vi "Initialise.vi"(8 "error in (no error)":errorcluster, 10 "Var Access":refnum<class "Var_Access.lvclass">[](array[class]), 11 "Var Bus in":refnum<class "Var Bus.lvclass">) -> (0 "error out":errorcluster, 3 "Var Bus out":refnum<class "Var Bus.lvclass">)   [LabVIEW 2021, in "Var Bus.lvclass"]
uses:
  Var Bus.lvclass
  Var Access/Var_Access.lvclass
  Var Bus.lvclass/Var Bus.ctl
  Properties/Write Var Access.vi
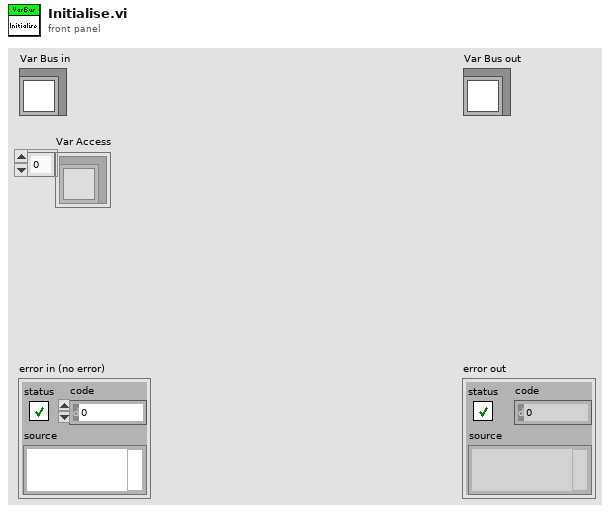
[diagram p1: front panel]
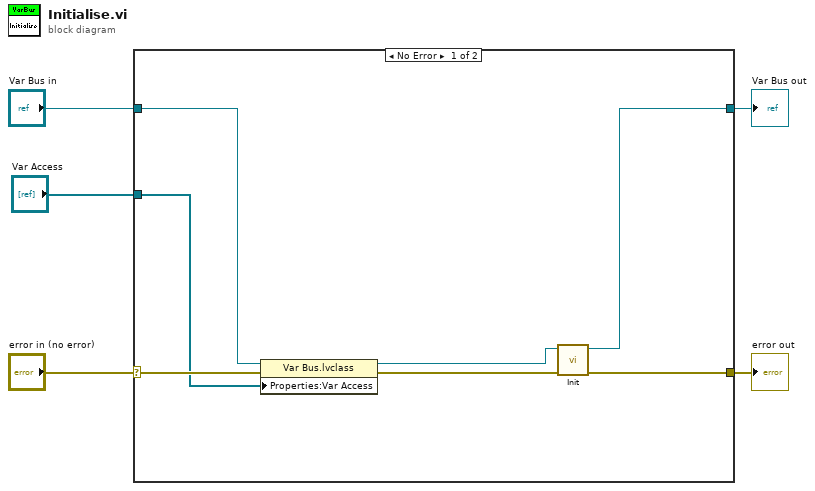
[diagram p0: block diagram]
diagram:
  n1 = case shown="No Error" "error in (no error)" {
    selector: "error in (no error)" -> [w10 w14]
    tunnel: [w12 w14] -> w4
    tunnel: [w11 w13] -> w2
    tunnel: "Var Bus in" -> [w9 w13]
    tunnel: "Var Access" -> [w8 _]
    frame No Error {
      n2 = property class="Var Bus.lvclass"(reference=w9, error in=w10, "Properties:Var Access"=w8) -> (reference out=w6:refnum<class "Var Bus.lvclass">, error out=w7:errorcluster)
      n3 = call-dynamic "Init.vi"("error in (no error)"=w7, "Data in"=w6) -> ("error out"=w12:errorcluster, "Data out"=w11:refnum<class "Var Bus.lvclass">)  [unwired: 8 in]
    }
    frame Error {
    }
  }
  "error out" <- w4
  "Var Bus out" <- w2
